vi "Vision Processing.vi"(4 "error in (no error)":errorcluster, 7 "Image Size":T3=enum."320x240") -> ()   [LabVIEW 2015]
uses:
  Vision Support Code/Camera Types.ctl
  <vilib>/Rock Robotics/WPI/Camera/WPI_CameraImageSize.ctl
  <vilib>/Rock Robotics/WPI/Camera/WPI_CameraWhite Balance Values.ctl
  <vilib>/Rock Robotics/WPI/Camera/WPI_CameraExposure Values.ctl
  <vilib>/Rock Robotics/WPI/Camera/WPI_CameraFrameRate.ctl
  Robot Global Data.vi
  <vilib>/vision/NI_Vision_Development_Module.lvlib
panel:
  in  "Flip Image":bool
  out "Width":dbl
  out "Highest Avg Score":dbl
  in  "Min Score Threshold":i32=75
  out "Detected Targets":T1(array[cluster]) {"Normalized Rect"."Numeric 5" format="%#_2g"; "Normalized Rect"."Numeric 3" format="%#_2g"; "Normalized Rect"."Numeric 2" format="%#_2g"; "Normalized Rect"."Numeric" format="%#_2g"}
  out "Sorted Particle Scores":T2(array[cluster]) {"Moment Factor" format="%#_3g"; "Aspect Ratio" format="%#_3g"; "Area to CH" format="%#_3g"; "X" format="%#_3g"; "Y" format="%#_3g"}
  in  "Display Original":bool=TRUE
  in  "Display Mask":bool=TRUE
  out "FPS":dbl
  in  "Emphasize Limit Tests":bool=TRUE
  in  "Camera Type":T4=enum."MS HD3000 square"
  in  "Aspect Fudge Factor":dbl=1.0
  in  "Score Threshold":dbl=75.0
  out "ms to process":u32
  out "Qualified Particles":i32
  in  "LED Color":T5={"Hue"={46.09028466854532, 182.57832914937742}, "Sat"={179.10714285714286, 255.0}, "Val"={194.28571428571428, 255.0}} {"Hue" scale=0.0..255.0 scale format="%#_3g"}
  out "Masked":T6(plugin-control)
  out "Original Image":T6(plugin-control)
  # "This is only the initial camera size.\nOther camera setup is done\non the diagram. Notice it is set\nonce before the loop but can be\nupdated within the loop if needed."
  # "Instructions:\nUse LED Color to threshold and build particles. Adjust calibration if needed.\nDisplays are very useful for debugging, but will slow down execution, so you\nmay want to disable once working.\nAnnotations show the rectangle and the scores from top to bottom.\nChange camera setting on diagram."
  # "Density Profile"
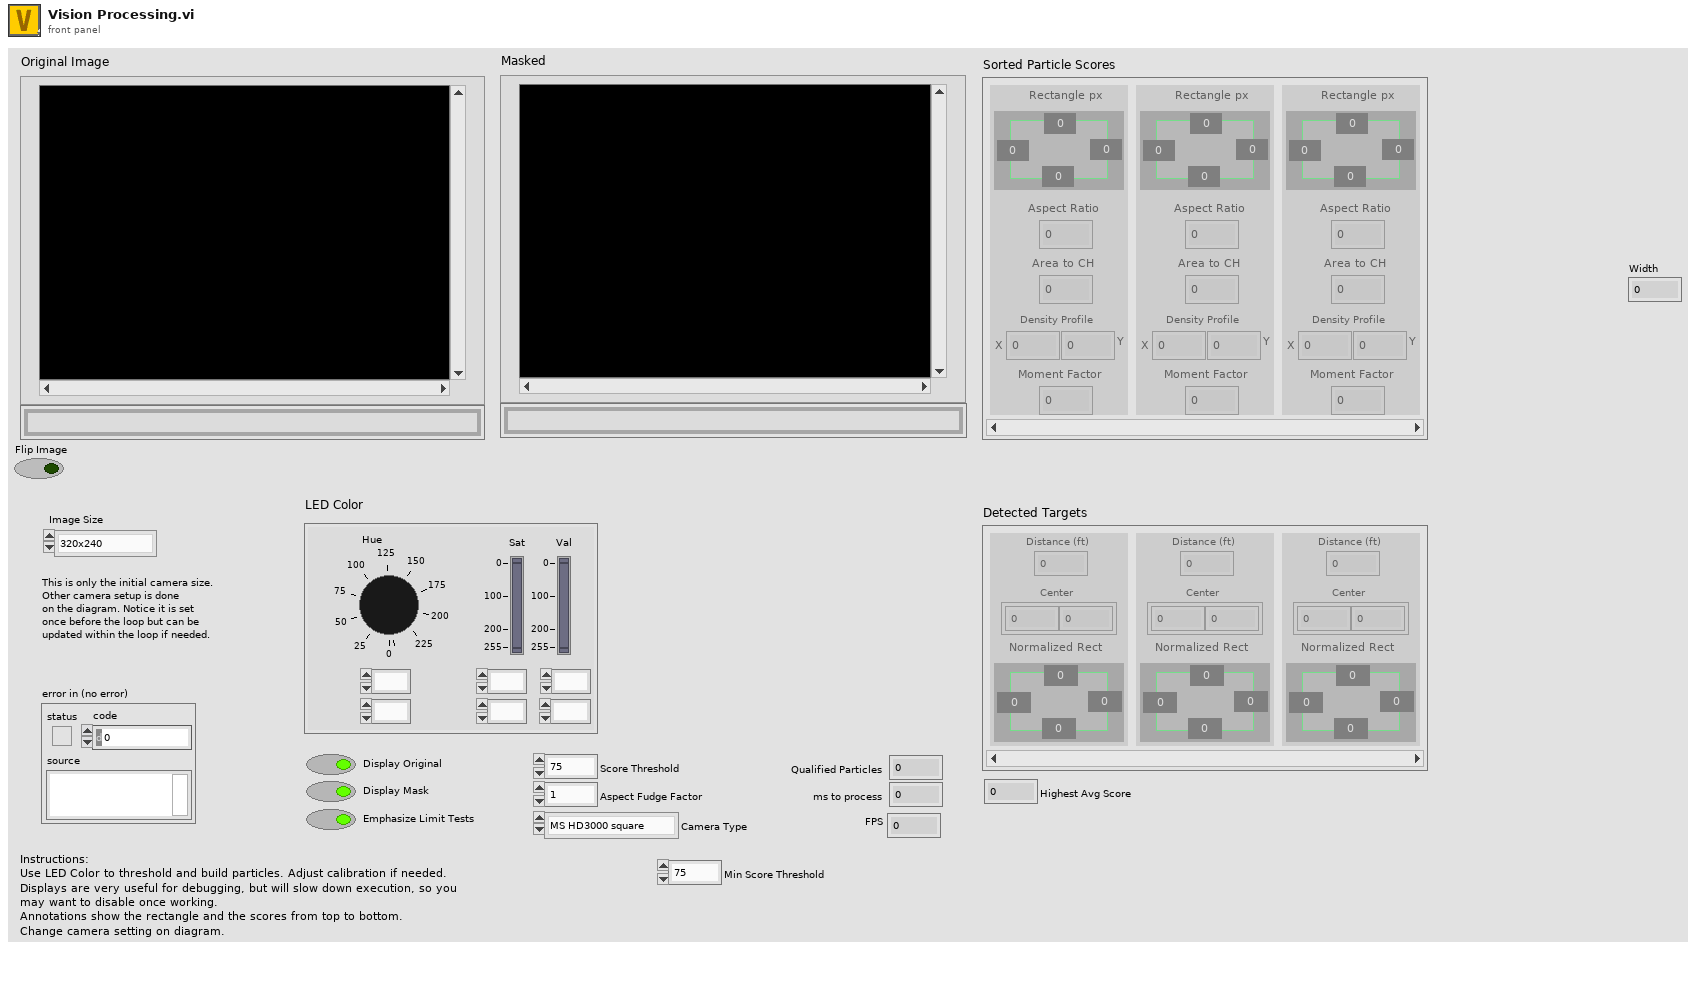
[diagram p1: front panel]
types:
  T1 = cluster{"Distance (ft)":dbl, "Center":cluster{dbl, dbl}, "Normalized Rect":cluster{"Numeric":dbl, "Numeric 2":dbl, "Numeric 3":dbl, "Numeric 5":dbl}}[]
  T2 = cluster{"Rectangle px":cluster{"Left":dbl, "Numeric 2":dbl, "Numeric 3":dbl, "Numeric 5":dbl}, "Aspect Ratio":dbl, "Area to CH":dbl, "X":dbl, "Y":dbl, "Moment Factor":dbl}[]
  T3 = typedef "WPI_CameraImageSize.ctl" = enum16{"640x480", "320x240", "160x120", "Custom"}
  T4 = typedef "Camera Types.ctl" = enum16{"206", "1011", "1013", "MS HD3000 square", "MS HD3000 640x480"}
  T5 = cluster{"Hue":cluster{dbl, dbl}, "Sat":cluster{dbl, dbl}, "Val":cluster{dbl, dbl}}
  T6 = typedef "IMAQ Image.ctl" = refnum<image>
  T7 = typedef "Image Type" = u32
  T8 = typedef "WPI_CameraFrameRate.ctl" = u32
  T9 = typedef "WPI_CameraExposure Values.ctl" = enum16{"Auto", "Flicker-free 50 Hz", "Flicker-free 60 Hz", "Hold current", "Custom"}
  T10 = typedef "WPI_CameraWhite Balance Values.ctl" = enum16{"Auto", "Fixed indoor", "Fixed outdoor 1", "Fixed outdoor 2", "Fixed fluorescent 1", "Fixed fluorescent 2", "Hold current", "Custom"}
  T11 = typedef "Particle Parameters" = i32
  T12 = typedef "WPI_CameraDevRef.ctl" = cluster{"Camera Address":string, "CameraStatus":errorcluster}
  T13 = cluster{"Rectangle":cluster{"Left":dbl, "Top":dbl, "Right":dbl, "Bottom":dbl}, "L":dbl, "Area to CH":dbl, "X":dbl, "Y":dbl, "Moment Factor":dbl}
  T14 = cluster{"Bounding box":cluster{"left":dbl, "top":dbl, "right":dbl, "bottom":dbl}, "Aspect Ratio":dbl, "Area to CH":dbl, "X Mask":dbl, "Y Mask":dbl, "Moment":dbl}[]
  T15 = cluster{"Rectangle":cluster{"Numeric":dbl, "Numeric 2":dbl, "Numeric 3":dbl, "Numeric 5":dbl}, "L":dbl, "Area to CH":dbl, "X":dbl, "Y":dbl, "Moment Factor":dbl}[]
  T16 = cluster{"Rectangle":cluster{"Numeric":dbl, "Numeric 2":dbl, "Numeric 3":dbl, "Numeric 5":dbl}, "L":dbl, "Area to CH":dbl, "X":dbl, "Y":dbl, "Moment Factor":dbl}
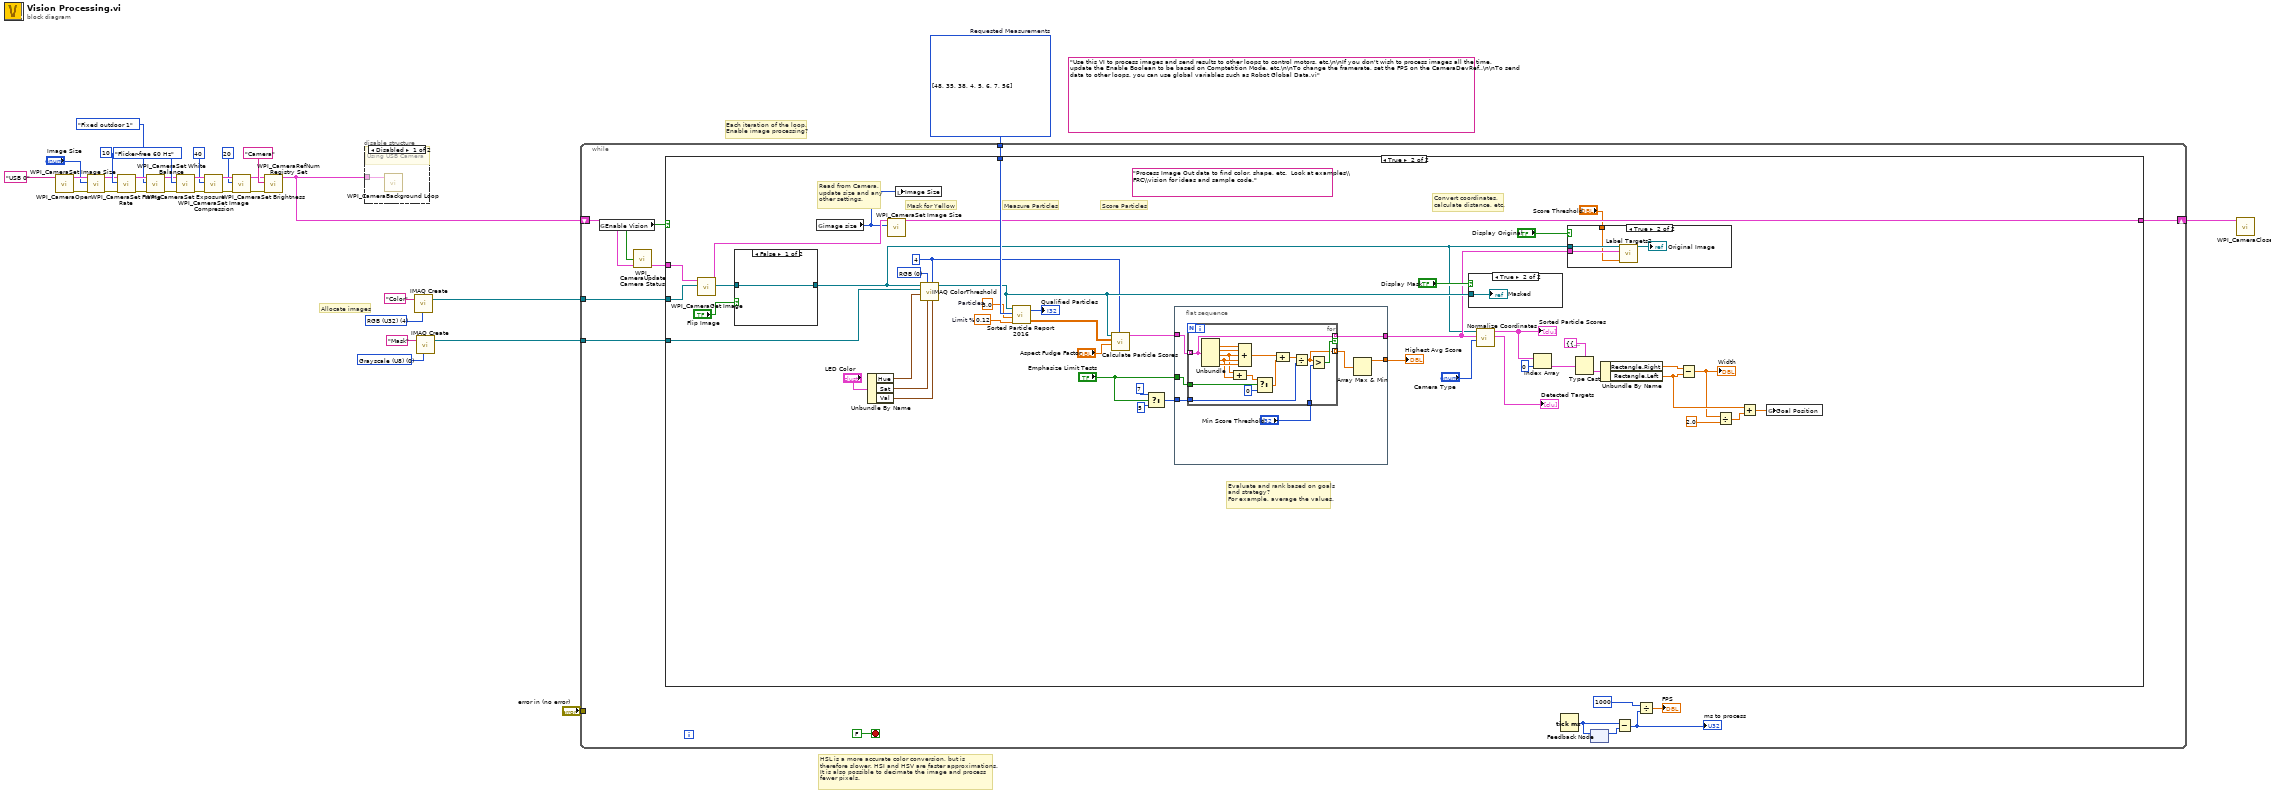
[diagram p0: block diagram]
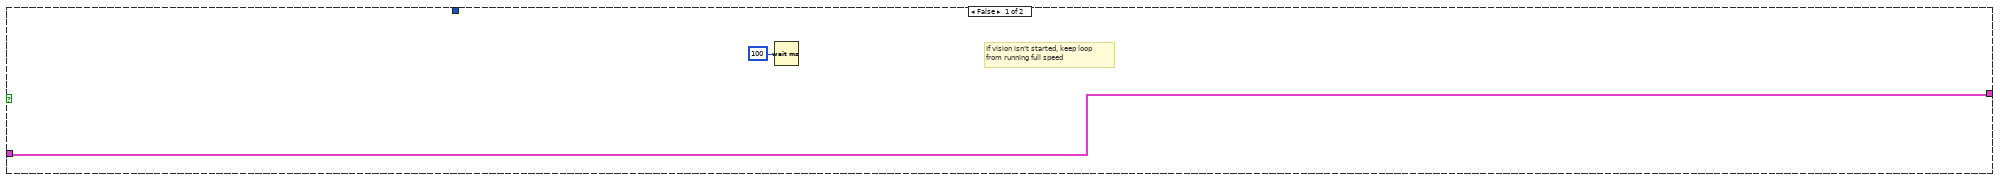
[diagram p3: hidden frame]
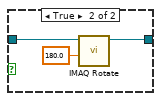
[diagram p4: hidden frame]
diagram:
  w2 = T7 0 items=["Grayscale (U8)", "Grayscale (I16)", "Grayscale (SGL)", "Complex (CSG)", "RGB (U32)", "HSL (U32)", "RGB (U64)", "Grayscale (U16)"] ("Image Type")
  (unwired) "Use this VI to process images and send results to other loops to control motors, etc.\n\nIf you don't wish to process images all the time, update the Enable Boolean to be based on Comptetition Mode, etc.\n\nTo change the framerate, set the FPS on the CameraDevRef..\n\nTo send data to other loops, you can use global variables such as Robot Global Data.vi"
  w31 = T7 4 items=["Grayscale (U8)", "Grayscale (I16)", "Grayscale (SGL)", "Complex (CSG)", "RGB (U32)", "HSL (U32)", "RGB (U64)", "Grayscale (U16)"] ("Image Type")
  w28 = T11[] [48, 35, 38, 4, 5, 6, 7, 56] items=["Center of Mass X", "Center of Mass Y", "First Pixel X", "First Pixel Y", "Bounding Rect Left", "Bounding Rect Top", "Bounding Rect Right", "Bounding Rect Bottom", "Max Feret Diameter Start X", "Max Feret Diameter Start Y", "Max Feret Diameter End X", "Max Feret Diameter End Y", "Max Horiz. Segment Length Left", "Max Horiz. Segment Length Right", "Max Horiz. Segment Length Row", "-", "Bounding Rect Width", "Bounding Rect Height", "Bounding Rect Diagonal", "Perimeter", "Convex Hull Perimeter", "Holes' Perimeter", "Max Feret Diameter", "Equivalent Ellipse Major Axis", "Equivalent Ellipse Minor Axis", "Equivalent Ellipse Minor Axis (Feret)", "Equivalent Rect Long Side", "Equivalent Rect Short Side", "Equivalent Rect Diagonal", "Equivalent Rect Short Side (Feret)", "Average Horiz. Segment Length", "Average Vert. Segment Length", "Hydraulic Radius", "Waddel Disk Diameter", "-", "Area", "Holes' Area", "Particle & Holes' Area", "Convex Hull Area", "Image Area", "-", "Number of Holes", "Number of Horiz. Segments", "Number of Vert. Segments", "-", "Orientation", "Max Feret Diameter Orientation", "-", "% Area/Image Area", "% Area/(Particle & Holes' Area)", "Ratio of Equivalent Ellipse Axes", "Ratio of Equivalent Rect Sides", "-", "Elongation Factor", "Compactness Factor", "Heywood Circularity Factor", "Type Factor", "-", "Sum X", "Sum Y", "Sum XX", "Sum XY", "Sum YY", "Sum XXX", "Sum XXY", "Sum XYY", "Sum YYY", "-", "Moment of Inertia XX", "Moment of Inertia XY", "Moment of Inertia YY", "Moment of Inertia XXX", "Moment of Inertia XXY", "Moment of Inertia XYY", "Moment of Inertia YYY", "Norm. Moment of Inertia XX", "Norm. Moment of Inertia XY", "Norm. Moment of Inertia YY", "Norm. Moment of Inertia XXX", "Norm. Moment of Inertia XXY", "Norm. Moment of Inertia XYY", "Norm. Moment of Inertia YYY", "Hu Moment 1", "Hu Moment 2", "Hu Moment 3", "Hu Moment 4", "Hu Moment 5", "Hu Moment 6", "Hu Moment 7"]  # Requested Measurements
  # "Each iteration of the loop,\nEnable image processing?"
  # "HSL is a more accurate color conversion, but is\ntherefore slower. HSI and HSV are faster approximations.\nIt is also possible to decimate the image and process\nfewer pixels."
  # "Allocate images"
  n1 = call <vilib>:"WPI_CameraOpen.vi"("Camera Address"="USB 0" ("format string")) -> ("error out"=w17:errorcluster, "CameraDevRef"=w16:T12)  [unwired: 1 in, 8 out]
  n2 = call <vilib>:"WPI_CameraSet Image Size.vi"("error in (no error)"=w17, "Image Size"="Image Size", "CameraDevRef"=w16) -> ("error out"=w18:errorcluster, "CameraDevRef Out"=w15:T12)  [unwired: 1 in, 6 out]
  n3 = call <vilib>:"WPI_CameraSet Frame Rate.vi"("error in (no error)"=w18, "Frame Rate (fps)"=T8 10, "CameraDevRef"=w15) -> ("error out"=w19:errorcluster, "CameraDevRef Out"=w13:T12)  [unwired: 7 out]
  n4 = call <vilib>:"WPI_CameraSet White Balance.vi"("error in (no error)"=w19, "White Balance"=WPI_CameraWhite_Balance_Values."Fixed outdoor 1", "CameraDevRef"=w13) -> ("error out"=w20:errorcluster, "CameraDevRef Out"=w14:T12)  [unwired: 1 in, 6 out]
  n5 = call <vilib>:"WPI_CameraSet Exposure.vi"("error in (no error)"=w20, "Exposure"=WPI_CameraExposure_Values."Flicker-free 60 Hz", "CameraDevRef"=w14) -> ("error out"=w21:errorcluster, "CameraDevRef Out"=w11:T12)  [unwired: 1 in, 6 out]
  n6 = call <vilib>:"WPI_CameraSet Image Compression.vi"("error in (no error)"=w21, "Compression"=40, "CameraDevRef"=w11) -> ("error out"=w22:errorcluster, "CameraDevRef Out"=w12:T12)  [unwired: 7 out]
  n7 = call <vilib>:"WPI_CameraSet Brightness.vi"("error in (no error)"=w22, "Brightness"=20, "CameraDevRef"=w12) -> ("error out"=w23:errorcluster, "CameraDevRef Out"=w6:T12)  [unwired: 7 out]
  n8 = call <vilib>:"WPI_CameraRefNum Registry Set.vi"("error in (no error)"=w23, "refnum name"="Camera", "CameraDevRef"=w6) -> ("CameraDevRef"=w3:T12)  [unwired: 1 in, 7 out]
  n9 = disable-structure shown="Disabled" {
    disable-tunnel: w3 -> [w33 _]
    frame Disabled {
      # "Using USB Camera"
      n10 = call <vilib>:"WPI_CameraBackground Loop.vi"("CameraDevRef"=w33) -> ()  [unwired: 11 in]
    }
    frame Enabled {
    }
  }
  n11 = call "IMAQ Create"("Image Name"="Color", "Image Type"=w31) -> ("New Image"=w30:T6)  [unwired: 2 in, 2 out]
  n12 = call "IMAQ Create"("Image Name"="Mask", "Image Type"=w2) -> ("New Image"=w1:T6)  [unwired: 2 in, 2 out]
  n13 = while {
    tunnel: w30 -> [w41]
    tunnel: w1 -> [w45]
    tunnel: w28 -> [w44]
    tunnel: "error in (no error)" -> [_]
    shift-right: [w37] -> w26
    shift-left: w3 -> [w39]
    stop <- FALSE stop-if-true
    n14 = global read "Robot Global Data.vi" "Enable Vision"() -> (w40:bool)
    n15 = call <vilib>:"WPI_CameraUpdate Camera Status.vi"("CameraDevRef In"=w39, "Enable Vision"=w40) -> ("CameraDevRef Out"=w38:T12)  [unwired: 3 in]
    n16 = case shown="True" w40 {
      tunnel: w45 -> [_ w50]
      tunnel: w44 -> [_ w93]
      tunnel: w38 -> [w47 w69]
      tunnel: w41 -> [_ w89]
      tunnel: [w47 w87] -> w37
      frame False {
        # "If vision isn't started, keep loop\nfrom running full speed"
        n17 = Wait (ms)(milliseconds to wait=u32 100) -> ()  [unwired: 1 out]
      }
      frame True {
        w72 = 4 ("Replace Value")
        w84 = u16 0 items=["RGB", "HSL", "HSV", "HSI"] ("Color Mode")
        (unwired) "Process Image Out data to find color, shape, etc.  Look at examples\\FRC\\vision for ideas and sample code."
        w90 = 0.12  # Limit %
        w92 = 3.0  # Particles
        # "Evaluate and rank based on goals\nand strategy?\nFor example, average the values."
        # "Read from Camera,\nupdate size and any\nother settings."
        # "Measure Particles"
        # "Convert coordinates,\ncalculate distance, etc."
        # "Score Particles"
        # "Mask for Yellow"
        n18 = call <vilib>:"WPI_CameraGet Image.vi"("Image"=w89, "CameraDevRef"=w69) -> ("Image Out"=w51:T6, "CameraDevRef Out"=w88:T12)  [unwired: 7 in, 1 out]
        n19 = case shown="False" "Flip Image" {
          tunnel: [w94 w96] -> w52
          tunnel: w51 -> [w94 w95]
          frame False {
          }
          frame True {
            n20 = call "IMAQ Rotate"("Angle (degrees)"=sgl 180.0, "Image Src"=w95) -> ("Image Dst Out"=w96:T6)  [unwired: 8 in, 1 out]
          }
        }
        n21 = global read "Robot Global Data.vi" "image size"() -> (w71:T3)
        n22 = Unbundle By Name("LED Color") -> ("Hue"=w67:cluster{dbl, dbl}, "Sat"=w66:cluster{dbl, dbl}, "Val"=w65:cluster{dbl, dbl})
        n23 = call <vilib>:"WPI_CameraSet Image Size.vi"("Image Size"=w71, "CameraDevRef"=w88) -> ("CameraDevRef Out"=w87:T12)  [unwired: 2 in, 7 out]
        n24 = local write "Image Size"(w71) -> ()
        n25 = call "IMAQ ColorThreshold"("Blue or Luma or Val or Inten Range"=w65, "Replace Value"=w72, "Green or Sat Range"=w66, "Color Mode"=w84, "Red or Hue Range"=w67, "Image Dst"=w50, "Image Src"=w52) -> ("Image Dst Out"=w83:T6)  [unwired: 3 in, 1 out]
        n26 = call "Sorted Particle Report 2016.vi"("Min Area Size %"=w90, "Particle Count Limit"=w92, "Pixel Measurements"=w93, "Image in"=w83) -> ("Sorted Data"=w82:dbl[][], "Particles"=→"Qualified Particles":i32)
        n27 = call "Calculate Particle Scores.vi"("Pixel Value"=w72, "Aspect Fudge Factor"="Aspect Fudge Factor", "Sorted Data"=w82, "Image in"=w83) -> ("Scores"=w80:T14)  [unwired: 7 in]
        n28 = Select(t=7, s="Emphasize Limit Tests", f=5) -> (s? t:f=w77:i32)
        n29 = flat-sequence {
          tunnel: w80 -> [w108]
          tunnel: w77 -> [w106]
          tunnel: [w109] -> w76
          tunnel: [w103] -> w74
          tunnel: "Emphasize Limit Tests" -> [w107]
          frame #0 {
            n30 = for {
              tunnel: w108 -> [w123] mode=indexing
              tunnel: [w123] -> w103 mode=indexing if=w122
              tunnel: [w121] -> w104 mode=indexing
              tunnel: w106 -> [w120]
              tunnel: "Min Score Threshold" -> [w119]
              tunnel: w107 -> [w112]
              n31 = Unbundle(w123) -> ("Aspect Ratio"=w125:dbl, "Area to CH"=w124:dbl, "X Mask"=w114:dbl, "Y Mask"=w115:dbl, "Moment"=w116:dbl)  [unwired: 1 out]
              n32 = Compound Arithmetic op=ADD(w114, w115) -> (w113:dbl)
              n33 = Compound Arithmetic op=ADD(w125, w124, w114, w115, w116) -> (w118:dbl)
              n34 = Select(t=w113, s=w112, f=0) -> (s? t:f=w111:dbl)
              n35 = Compound Arithmetic op=ADD(w118, w111) -> (w117:dbl)
              n36 = Divide(x=w117, y=w120) -> (x/y=w121:dbl)
              n37 = Greater?(x=w121, y=w119) -> (0:w122:bool)
            }
            n38 = Array Max & Min(array=w104) -> (max value=w109:dbl)  [unwired: 3 out]
          }
        }
        n39 = case shown="True" "Display Mask" {
          tunnel: w83 -> [_ w102]
          frame False {
          }
          frame True {
            "Masked" <- w102
          }
        }
        n40 = call "Normalize Coordinates.vi"("Camera Type"="Camera Type", "Targets"=w74, "Image in"=w52) -> ("Found Targets"=→"Detected Targets":T1, "Sorted Scores"=w64:T15)  [unwired: 7 in]
        "Sorted Particle Scores" <- w64
        n41 = Index Array(array=w64, index=0) -> (element=w61:T16)
        n42 = case shown="True" "Display Original" {
          tunnel: w52 -> [_ w101]
          tunnel: w74 -> [_ w99]
          tunnel: "Score Threshold" -> [_ w98]
          frame False {
          }
          frame True {
            n43 = call "Label Targets2.vi"("Score Threshold"=w98, "Targets"=w99, "Image in"=w101) -> ("Image out"=→"Original Image":T6)  [unwired: 8 in]
          }
        }
        n44 = Type Cast(type=T13 {"Rectangle"={"Left"=0.0, "Top"=0.0, "Right"=0.0, "Bottom"=0.0}, "L"=0.0, "Area to CH"=0.0, "X"=0.0, "Y"=0.0, "Moment Factor"=0.0} ("element"), x=w61) -> (*(type *) &x=w60:T13)
        n45 = Unbundle By Name(w60) -> ("Rectangle.Right"=w56:dbl, "Rectangle.Left"=w57:dbl)
        n46 = Subtract(x=w56, y=w57) -> (x-y=w55:dbl)
        "Width" <- w55
        n47 = Divide(x=w55, y=2.0) -> (x/y=w54:dbl)
        n48 = Add(x=w57, y=w54) -> (x+y=w53:dbl)
        n49 = global write "Robot Global Data.vi" "Goal Position"(w53) -> ()
        "Highest Avg Score" <- w76
      }
    }
    n50 = Tick Count (ms)() -> (millisecond timer value=w42:u32)
    n51 = feedback-in #1(w42) -> ()
    n52 = feedback #1() -> (w43:u32)  [unwired: 1 in]
    n53 = Subtract(x=w42, y=w43) -> (x-y=w34:u32)
    "ms to process" <- w34
    n54 = Divide(x=1000 ("Brightness"), y=w34) -> (x/y=→"FPS":dbl)
  }
  n55 = call <vilib>:"WPI_CameraClose.vi"("CameraDevRef"=w26) -> ()  [unwired: 1 in, 10 out]
